vi "Spartan HTTP Valid HTTP Config.vi"(8 "error in (no error)":errorcluster) -> (0 "error out":errorcluster, 2 "problem description":string, 3 "valid":bool)   [LabVIEW 2011]
uses:
  ITK EXT/http/http0.llb/HTTP Config.ctl
  ITK EXT/http/http0.llb/HTTP LVHTTP Global.vi
  ITK EXT/http/image.llb/HTTP Panel Image.glb
  ITK EXT/http/config.llb/HTTP SRM.vi
panel:
  out "duplicate config":T1
  in  "config":T1
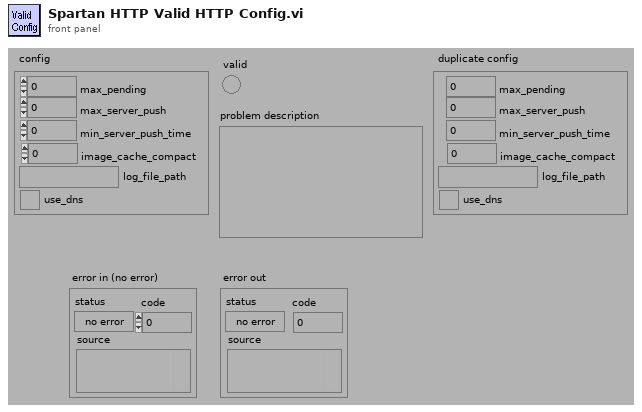
[diagram p1: front panel]
types:
  T1 = typedef "HTTP Config.ctl" = cluster{"max_pending":i32, "max_server_push":i32, "min_server_push_time":i32, "log_file_path":path, "use_dns":bool, "image_cache_compact":i32}
  T2 = cluster{"msg":string, "srvr":bool, "rsrc":bool, "warning":bool}[]
  T3 = enum32{"MaxPending", "MaxServerPush", "StartServers", "DocumentRoot", "LVhttpLog"}
  T4 = cluster{"Max":i32, "MinTime":i32, "Refresh":dbl, "LifeSpan":i32}
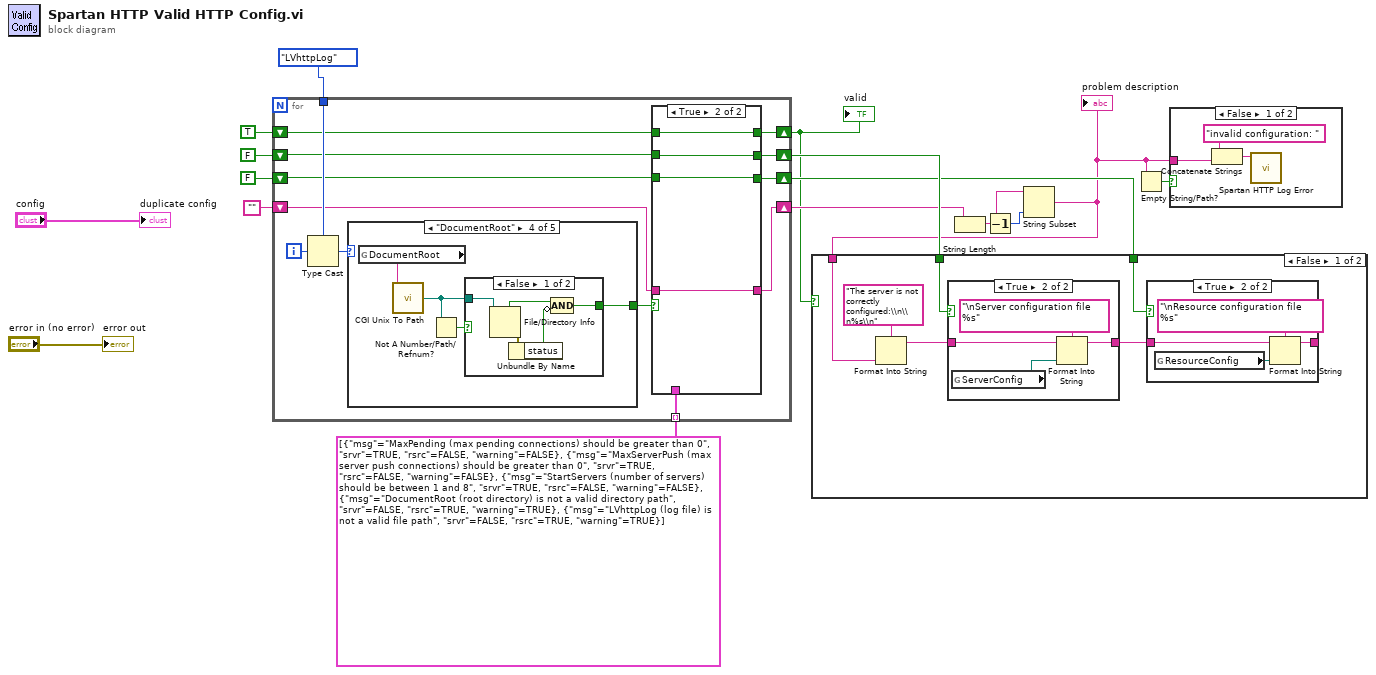
[diagram p0: block diagram]
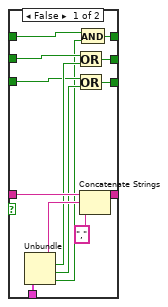
[diagram p6: hidden frame]
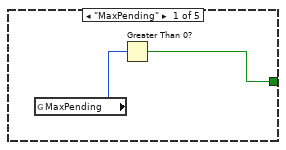
[diagram p7: hidden frame]
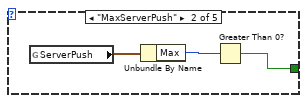
[diagram p8: hidden frame]
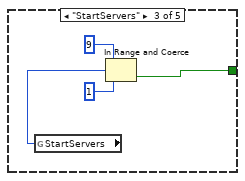
[diagram p9: hidden frame]
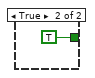
[diagram p10: hidden frame]
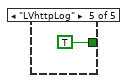
[diagram p11: hidden frame]
diagram:
  n1 = for {
    shift-right: [w23] -> w7
    shift-left: "" -> [w25]
    tunnel: T3."LVhttpLog" -> [w27]
    tunnel: T2 [{"msg"="MaxPending (max pending connections) should be greater than 0", "srvr"=TRUE, "rsrc"=FALSE, "warning"=FALSE}, {"msg"="MaxServerPush (max server push connections) should be greater than 0", "srvr"=TRUE, "rsrc"=FALSE, "warning"=FALSE}, {"msg"="StartServers (number of servers) should be between 1 and 8", "srvr"=TRUE, "rsrc"=FALSE, "warning"=FALSE}, {"msg"="DocumentRoot (root directory) is not a valid directory path", "srvr"=FALSE, "rsrc"=TRUE, "warning"=TRUE}, {"msg"="LVhttpLog (log file) is not a valid file path", "srvr"=FALSE, "rsrc"=TRUE, "warning"=TRUE}] -> [w24] mode=indexing
    shift-right: [w22] -> w9
    shift-left: FALSE -> [w21]
    shift-right: [w20] -> w8
    shift-left: FALSE -> [w19]
    shift-right: [w18] -> w3
    shift-left: TRUE -> [w17]
    i -> [w29]
    n2 = Type Cast(type=w27, x=w29) -> (*(type *) &x=w28:T3)
    n3 = case shown="\"DocumentRoot\"" w28 {
      tunnel: [w49 w52 w54 w60 TRUE] -> w26
      frame "MaxPending" {
        n4 = global read "HTTP LVHTTP Global.vi" "MaxPending"() -> (w48:i32)
        n5 = Greater Than 0?(x=w48) -> (x > 0?=w49:bool)
      }
      frame "MaxServerPush" {
        n6 = global read "HTTP Panel Image.glb" "ServerPush"() -> (w51:T4)
        n7 = Unbundle By Name(w51) -> ("Max"=w50:i32)
        n8 = Greater Than 0?(x=w50) -> (x > 0?=w52:bool)
      }
      frame "StartServers" {
        n9 = global read "HTTP LVHTTP Global.vi" "StartServers"() -> (w53:i32)
        n10 = In Range and Coerce(upper limit=9 ("lo"), x=w53, lower limit=1 ("lo")) -> (In Range?=w54:bool)  [unwired: 1 out]
      }
      frame "DocumentRoot" {
        n11 = global read "HTTP SRM.vi" "DocumentRoot"() -> (w57:string)
        n12 = call "CGI Unix To Path.vi"("unix path"=w57) -> ("platform path"=w58:path)  [unwired: 1 out]
        n13 = Not A Number/Path/Refnum?(number/path/refnum=w58) -> (NaN/Path/Refnum?=w59:bool)
        n14 = case shown="False" w59 {
          tunnel: w58 -> [w65 _]
          tunnel: [w64 TRUE] -> w60
          frame False {
            n15 = File/Directory Info(path=w65) -> (directory=w63:bool, error out=w61:errorcluster)  [unwired: 1 in, 5 out]
            n16 = Unbundle By Name(w61) -> ("status"=w62:bool)
            n17 = Compound Arithmetic op=AND(w63, invert w62) -> (w64:bool)
          }
          frame True {
          }
        }
      }
      frame "LVhttpLog" {
      }
    }
    n18 = case shown="True" w26 {
      tunnel: w25 -> [w43 w47]
      tunnel: w24 -> [w41 _]
      tunnel: [w42 w47] -> w23
      tunnel: [w39 w46] -> w22
      tunnel: w21 -> [w38 w46]
      tunnel: [w36 w45] -> w20
      tunnel: w19 -> [w35 w45]
      tunnel: [w31 w44] -> w18
      tunnel: w17 -> [w30 w44]
      frame False {
        n19 = Unbundle(w41) -> ("msg"=w40:string, "srvr"=w37:bool, "rsrc"=w34:bool, "warning"=w32:bool)
        n20 = Or(x=w38, y=w37) -> (x .or. y?=w39:bool)
        n21 = Or(x=w35, y=w34) -> (x .or. y?=w36:bool)
        n22 = And(x=w30, y=w32) -> (x .and. y?=w31:bool)
        n23 = Concatenate Strings(w43, w40, ",") -> (w42:string)
      }
      frame True {
      }
    }
  }
  "valid" <- w3
  n24 = String Length(string=w7) -> (length=w6:i32)
  n25 = Decrement(x=w6) -> (x-1=w5:i32)
  n26 = String Subset(string=w7, length (rest)=w5) -> (substring=w1:string)  [unwired: 1 out]
  "problem description" <- w1
  n27 = case shown="False" w3 {
    tunnel: w1 -> [w72 _]
    tunnel: w9 -> [w70 _]
    tunnel: w8 -> [w68 _]
    frame False {
      n28 = Format Into String(format string="The server is not correctly configured:\\n\\n%s\\n", w72) -> (resulting string=w71:string)  [unwired: 2 in, 1 out]
      n29 = case shown="True" w70 {
        tunnel: w71 -> [w79 w83]
        tunnel: [w79 w80] -> w69
        frame False {
        }
        frame True {
          n30 = global read "HTTP LVHTTP Global.vi" "ServerConfig"() -> (w81:path)
          n31 = Format Into String(format string="\nServer configuration file %s", initial string=w83, w81) -> (resulting string=w80:string)  [unwired: 1 in, 1 out]
        }
      }
      n32 = case shown="True" w68 {
        tunnel: w69 -> [w74 w78]
        tunnel: [w74 w75] -> _
        frame False {
        }
        frame True {
          n33 = global read "HTTP LVHTTP Global.vi" "ResourceConfig"() -> (w76:path)
          n34 = Format Into String(format string="\nResource configuration file %s", initial string=w78, w76) -> (resulting string=w75:string)  [unwired: 1 in, 1 out]
        }
      }
    }
    frame True {
    }
  }
  n35 = Empty String/Path?(string/path=w1) -> (empty?=w2:bool)
  n36 = case shown="False" w2 {
    tunnel: w1 -> [w86 _]
    frame False {
      n37 = Concatenate Strings("invalid configuration: " ("message"), w86) -> (w84:string)
      n38 = call "Spartan HTTP Log Error.vi"("message"=w84) -> ()  [unwired: 2 in, 5 out]
    }
    frame True {
    }
  }
  "duplicate config" <- "config"
  "error out" <- "error in (no error)"
